vi "P17b_Buffer_Out.vi"() -> ()   [LabVIEW 2022 SP3]
panel:
  in  "Boolean":bool
  in  "stop":bool
  # "P17b_Buffer_Out"
  # "Equipo C\nJairo Issac García López\nRodolfo Durón Hernandez\nRoberto Carlos Herrera Pérez\nSebastián Rodríguez Posada"
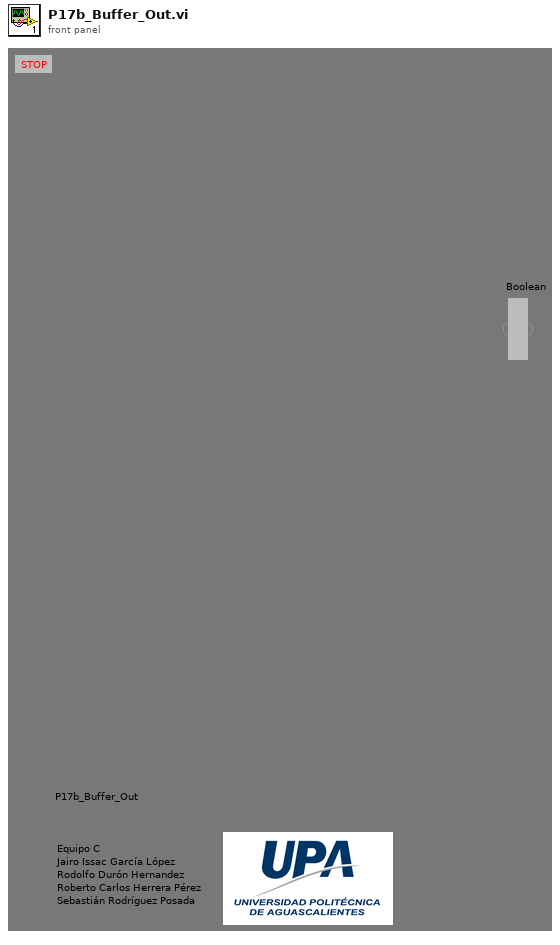
[diagram p1: front panel]
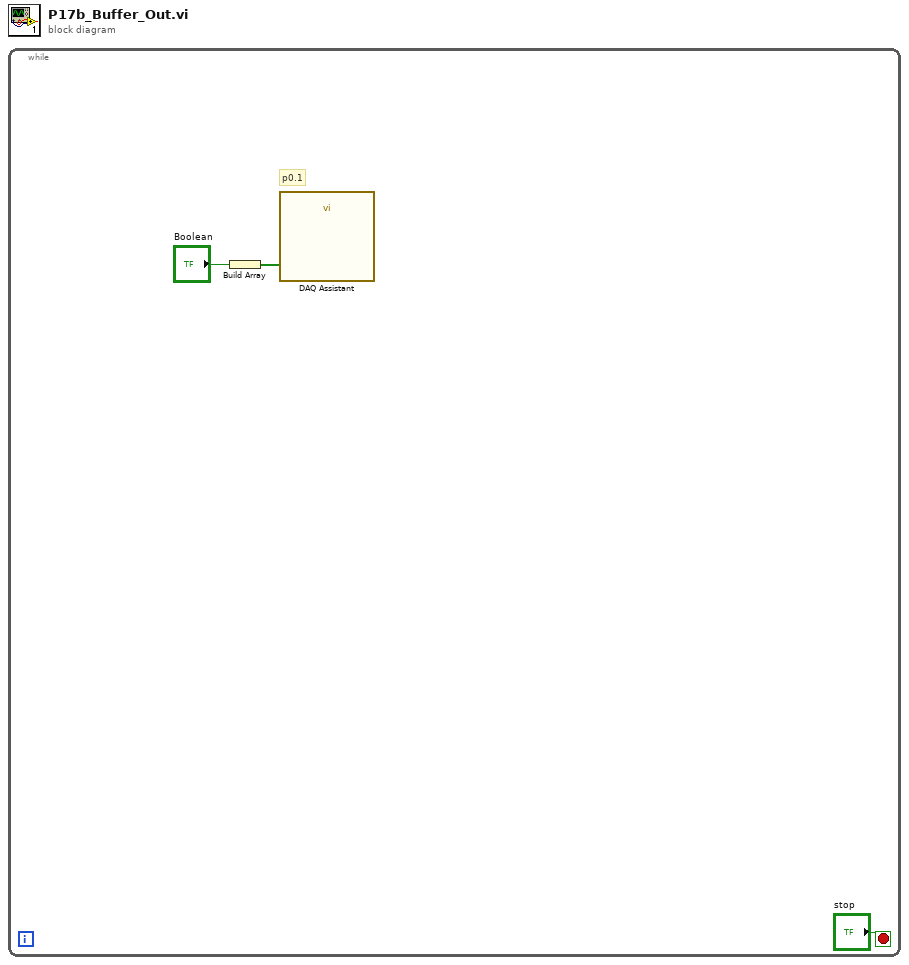
[diagram p0: block diagram]
diagram:
  n1 = while {
    stop <- "stop" stop-if-true
    # "p0.1"
    n2 = Build Array("Boolean") -> (w1:bool[])
    n3 = call "DAQ Assistant"("data"=w1) -> ()  [unwired: 17 in, 2 out]
  }
